vi "DataLogger.LogData.vi"(8 "error in (no error)":errorcluster, 9 "Value":string, 10 "DIM Service":string, 11 "i ref in":refnum<vi>) -> (0 "error out":errorcluster, 3 "i ref out":refnum<vi>)   [LabVIEW 2014, in "DataLogger.lvlib"]
uses:
  DataLogger.lvlib
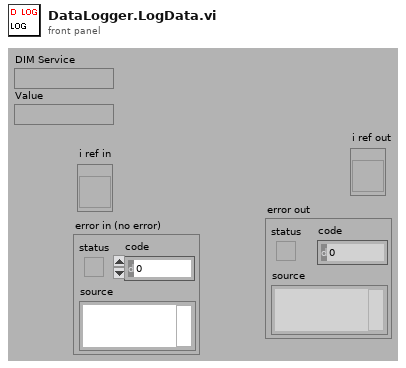
[diagram p1: front panel]
types:
  T1 = enum16{"open", "replace", "create", "open or create", "replace or create", "replace or create with confirmation"}
  T2 = typedef "DataLogger.lvlib/DataLogger.i attribute.ctl" = cluster{"Service Names":string[], "Path":string[], "Service Alarm Index":i32[], "Service Alarm Limit1":dbl[], "Service Alarm Limit2":dbl[], "Service Alarm Indicator":bool[], "alarmID":i32, "pathID":i32, "SoundDeviceID":i32, "SoundFile":string, "SoundID":i32, "SoundFileID":i32}
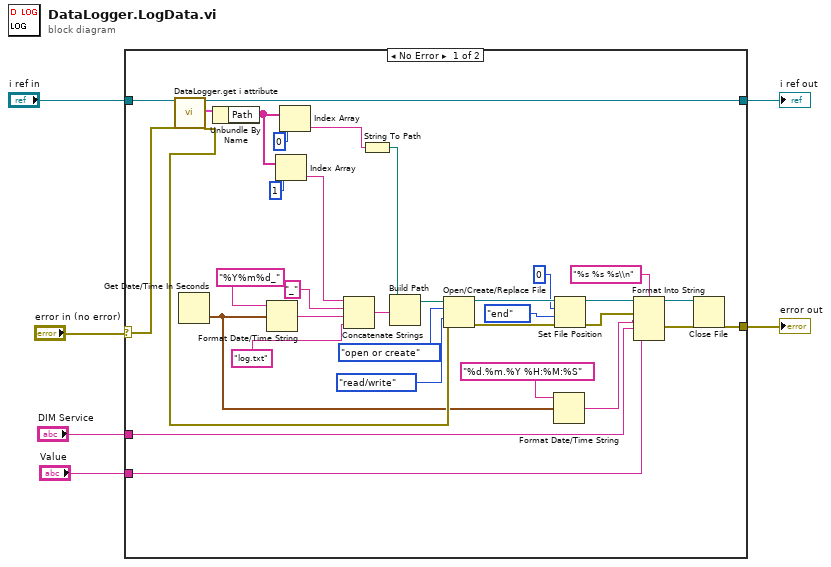
[diagram p0: block diagram]
diagram:
  n1 = case shown="No Error" "error in (no error)" {
    selector: "error in (no error)" -> [w35 w41]
    tunnel: "i ref in" -> [w36 w42]
    tunnel: [w34 w42] -> w4
    tunnel: [w29 w41] -> w3
    tunnel: "DIM Service" -> [w12 _]
    tunnel: "Value" -> [w11 _]
    frame No Error {
      n2 = call "DataLogger.get i attribute.vi"("i ref in"=w36, "error in (no error)"=w35) -> ("i ref out"=w34:refnum<vi>, "i attribute"=w33:T2, "error out"=w24:errorcluster)  [unwired: 15 in]
      n3 = Get Date/Time In Seconds() -> (seconds since 1Jan1904=w15:timestamp)
      n4 = Unbundle By Name(w33) -> ("Path"=w9:string[])
      n5 = Format Date/Time String(time format string (%c)="%Y%m%d_", seconds (now)=w15) -> (date/time string=w38:string)  [unwired: 1 in]
      n6 = Index Array(array=w9, index=1 ("length")) -> (element=w7:string)
      n7 = Index Array(array=w9, index=0 ("length")) -> (element=w27:string)
      n8 = Concatenate Strings(w7, "_" ("string"), w38, "log.txt" ("string")) -> (w40:string)
      n9 = String To Path(string=w27) -> (path=w26:path)
      n10 = Build Path(base path=w26, name or relative path=w40) -> (appended path=w22:path)
      n11 = Open/Create/Replace File(file path (use dialog)=w22, error in=w24, operation (0:open)=T1."open or create", access (0:read/write)=enum16{"read/write", "read-only", "write-only"}."read/write") -> (refnum out=w21:refnum<file>, error out=w20:errorcluster)  [unwired: 2 in, 1 out]
      n12 = Format Date/Time String(time format string (%c)="%d.%m.%Y %H:%M:%S", seconds (now)=w15) -> (date/time string=w13:string)  [unwired: 1 in]
      n13 = Set File Position(offset (in bytes) (0)=i64 0, refnum=w21, from (0:start)=enum16{"start", "end", "current"}."end", error in=w20) -> (refnum out=w18:refnum<file>, error out=w19:errorcluster)
      n14 = Format Into String(format string="%s %s %s\\n", initial string=w18, error in=w19, w13, w12, w11) -> (resulting string=w30:refnum<file>, error out=w31:errorcluster)
      n15 = Close File(refnum=w30, error in=w31) -> (error out=w29:errorcluster)  [unwired: 1 out]
    }
    frame Error {
    }
  }
  "error out" <- w3
  "i ref out" <- w4
